vi "1 Ball Side.vi"(1 "Run?":bool) -> ()   [LabVIEW 2013]
uses:
  Globals/Homes.vi
  Globals/Useful Values.vi
panel:
  out "Fire":bool
  out "Ready for Vision?":bool
  out "Done?":bool
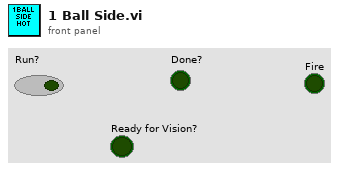
[diagram p1: front panel]
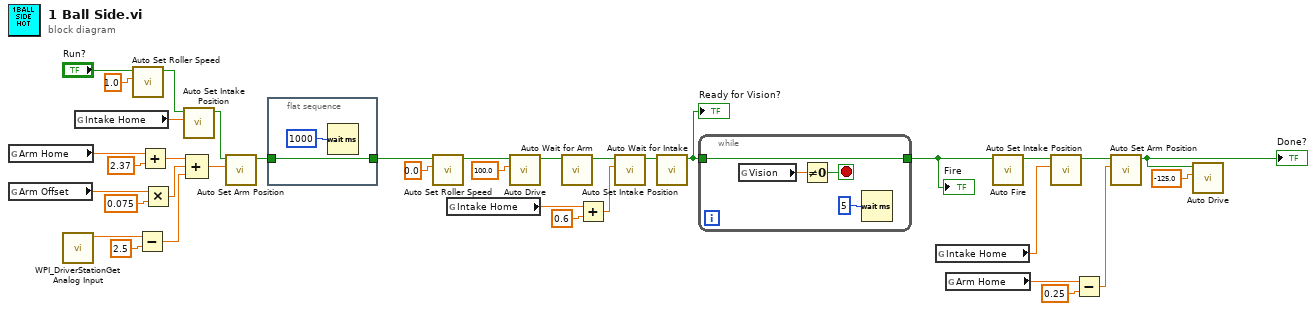
[diagram p0: block diagram]
diagram:
  n1 = global read "Homes.vi" "Arm Home"() -> (w14:dbl)
  n2 = global read "Useful Values.vi" "Arm Offset"() -> (w11:dbl)
  n3 = call <vilib>:"WPI_DriverStationGet Analog Input.vi"() -> ("Analog 1 (V)"=w8:dbl)  [unwired: 8 in, 3 out]
  n4 = global read "Homes.vi" "Intake Home"() -> (w30:dbl)
  n5 = call "Auto Set Roller Speed.vi"("Value"=1.0, "Run?"="Run?") -> ("Done"=w23:bool)  [unwired: 9 in]
  n6 = Subtract(x=w8, y=2.5) -> (x-y=w7:dbl)
  n7 = Add(x=w14, y=2.37) -> (x+y=w10:dbl)
  n8 = Multiply(x=w11, y=0.075) -> (x*y=w13:dbl)
  n9 = call "Auto Set Intake Position.vi"("Intake Position"=w30, "Run?"=w23) -> ("Done"=w16:bool)  [unwired: 9 in]
  n10 = Compound Arithmetic op=ADD(w10, w13, w7) -> (w6:dbl)
  n11 = call "Auto Set Arm Position.vi"("Arm Position"=w6, "Run?"=w16) -> ("Done"=w17:bool)  [unwired: 9 in]
  n12 = flat-sequence {
    tunnel: w17 -> [w38]
    tunnel: [w38] -> w21
    frame #0 {
      n13 = Wait (ms)(milliseconds to wait=u32 1000) -> ()  [unwired: 1 out]
    }
  }
  n14 = call "Auto Set Roller Speed.vi"("Value"=0.0, "Run?"=w21) -> ("Done"=w5:bool)  [unwired: 9 in]
  n15 = global read "Homes.vi" "Intake Home"() -> (w31:dbl)
  n16 = call "Auto Drive.vi"("Amount"=100.0, "Run?"=w5) -> ("Done"=w19:bool)  [unwired: 9 in]
  n17 = call "Auto Wait for Arm.vi"("Run?"=w19) -> ("Done"=w20:bool)  [unwired: 10 in]
  n18 = Add(x=w31, y=0.6) -> (x+y=w35:dbl)
  n19 = call "Auto Set Intake Position.vi"("Intake Position"=w35, "Run?"=w20) -> ("Done"=w22:bool)  [unwired: 9 in]
  n20 = call "Auto Wait for Intake.vi"("Run?"=w22) -> ("Done"=w2:bool)  [unwired: 10 in]
  "Ready for Vision?" <- w2
  n21 = while {
    tunnel: w2 -> [w39]
    tunnel: [w39] -> w3
    stop <- w42 stop-if-true
    n22 = global read "Useful Values.vi" "Vision"() -> (w41:dbl)
    n23 = Not Equal To 0?(x=w41) -> (x != 0?=w42:bool)
    n24 = Wait (ms)(milliseconds to wait=u32 5) -> ()  [unwired: 1 out]
  }
  "Fire" <- w3
  n25 = global read "Homes.vi" "Intake Home"() -> (w29:dbl)
  n26 = global read "Homes.vi" "Arm Home"() -> (w27:dbl)
  n27 = call "Auto Fire.vi"("Run?"=w3) -> ("Done"=w34:bool)  [unwired: 10 in]
  n28 = call "Auto Set Intake Position.vi"("Intake Position"=w29, "Run?"=w34) -> ("Done"=w33:bool)  [unwired: 9 in]
  n29 = Subtract(x=w27, y=0.25) -> (x-y=w28:dbl)
  n30 = call "Auto Set Arm Position.vi"("Arm Position"=w28, "Run?"=w33) -> ("Done"=w1:bool)  [unwired: 9 in]
  "Done?" <- w1
  n31 = call "Auto Drive.vi"("Amount"=-125.0, "Run?"=w1) -> ()  [unwired: 9 in, 1 out]
